vi "get value of int32 pointer.vi"(8 "error in (no error)":errorcluster, 11 "pointer in":u64) -> (0 "error out":errorcluster, 2 "value":i32, 3 "pointer out":u64)   [LabVIEW 2013, in "Linux Errno.lvlib"]
uses:
  Linux Errno.lvlib
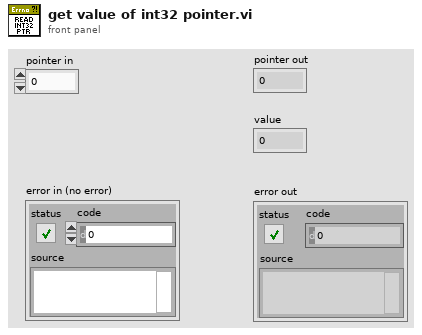
[diagram p1: front panel]
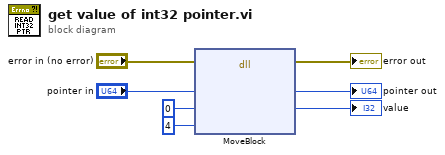
[diagram p0: block diagram]
diagram:
  n1 = dll-call lib="LabVIEW" fn="MoveBlock"(error in="error in (no error)", "pointer"="pointer in", "data"=0, "size"=u64 4) -> (error out=→"error out":errorcluster, "pointer"=→"pointer out":u64, "data"=→"value":i32)  [unwired: 4 in, 1 out]
